vi "Configure Scale Band IO.vi"(0 "VISA resource name":refnum<visa-resource-name>, 1 "Lower Position (In Log Calc) (1.00E+0)":dbl=1.0 format="%.2e", 2 "Upper Position (In Log Calc) (1.00E+2)":dbl=100.0 format="%.2e", 5 "Channel (0001)":string="0001", 7 "Area (0 : Off)":i32(ring) items=["Off", "In", "Out"], 9 "Color":cluster{"R":i32, "G":i32, "B":i32} {"B" min=0 max=255 step=1; "G" min=0 max=255 step=1; "R" min=0 max=255 step=1}, 11 "error in (no error)":errorcluster, 12 "Lower Position (0)":i32, 13 "Upper Position (1)":i32=1) -> (4 "VISA resource name out":refnum<visa-resource-name>, 6 "Channel":string, 15 "error out":errorcluster)   [LabVIEW 2020, in "Yokogawa GX Series.lvlib"]
doc: "Sets the green band of IO channel.\n\nCommand: SBandIO"
uses:
  <instrlib>/Yokogawa GX Series/Yokogawa GX Series.lvlib
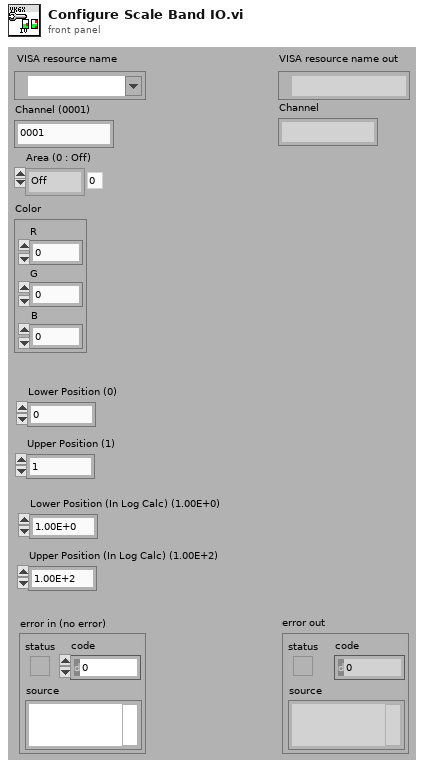
[diagram p1: front panel]
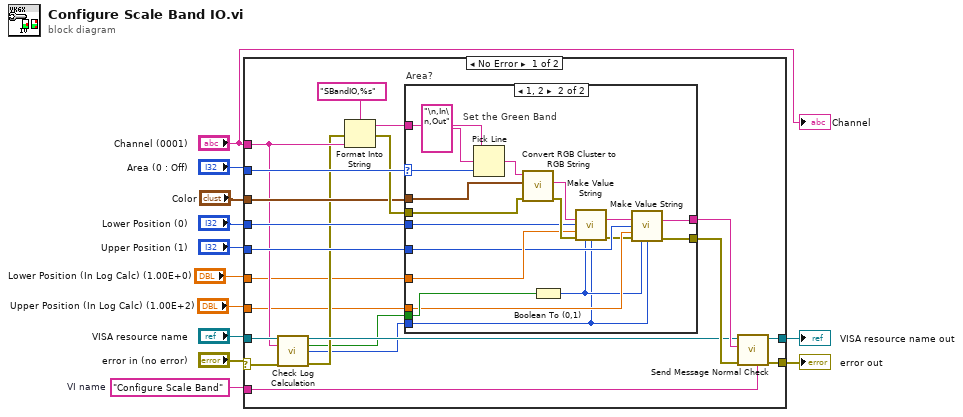
[diagram p0: block diagram]
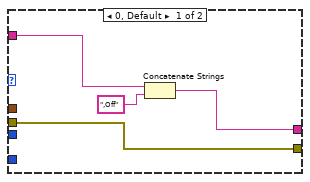
[diagram p2: hidden frame]
diagram:
  w12 = "Configure Scale Band"  # VI name
  n1 = case shown="No Error" "error in (no error)" {
    selector: "error in (no error)" -> [w21 w57]
    tunnel: w12 -> [w32 _]
    tunnel: "Area (0 : Off)" -> [w31 _]
    tunnel: "Lower Position (0)" -> [w28 _]
    tunnel: "Upper Position (1)" -> [w27 _]
    tunnel: "VISA resource name" -> [w20 w58]
    tunnel: [w24 w58] -> w7
    tunnel: [w23 w57] -> w6
    tunnel: "Color" -> [w22 _]
    tunnel: "Channel (0001)" -> [w19 _]
    tunnel: "Lower Position (In Log Calc) (1.00E+0)" -> [w16 _]
    tunnel: "Upper Position (In Log Calc) (1.00E+2)" -> [w15 _]
    frame No Error {
      n2 = call <instrlib>:"Check Log Calculation.vi"("VISA resource name"=w20, "Channel (0001)"=w19, "error in (no error)"=w21) -> ("VISA resource name out"=w18:refnum<visa-resource-name>, "Result"=w14:bool, "Float Position"=w13:i32, "error out"=w17:errorcluster)  [unwired: 9 in]
      n3 = Format Into String(format string="SBandIO,%s", error in=w17, w19) -> (resulting string=w26:string, error out=w30:errorcluster)  [unwired: 1 in]
      n4 = case "Area?" shown="1, 2" w31 {
        selector: w31 -> [_ w55]
        tunnel: w30 -> [w37 w52]
        tunnel: [w37 w41] -> w29
        tunnel: w28 -> [_ w48]
        tunnel: w27 -> [_ w44]
        tunnel: [w34 w40] -> w25
        tunnel: w26 -> [w35 w54]
        tunnel: w22 -> [_ w53]
        tunnel: w16 -> [_ w47]
        tunnel: w15 -> [_ w43]
        tunnel: w14 -> [_ w46]
        tunnel: w13 -> [_ w38]
        frame 0, Default {
          n5 = Concatenate Strings(w35, ",Off") -> (w34:string)
        }
        frame 1, 2 {
          # "Set the Green Band"
          n6 = Pick Line(string ("")=w54, multi-line string="\n,In\n,Out" ("形式文字列"), line index=w55) -> (output string=w51:string)
          n7 = call <instrlib>:"Convert RGB Cluster to RGB String.vi"("error in (no error)"=w52, "RGB"=w53, "Initial String"=w51) -> ("error out"=w50:errorcluster, "RGB String"=w49:string)  [unwired: 7 in]
          n8 = Boolean To (0,1)(Boolean=w46) -> (0, 1=w39:i16)
          n9 = call <instrlib>:"Make Value String.vi"("Initial String (\"\")"=w49, "Int Value (0)"=w48, "Float Value (0)"=w47, "Error In"=w50, "Kind Of Value (0: Int)"=w39, "Float Decimal Position (1)"=w38) -> ("Resulting String"=w45:string, "Error Out"=w42:errorcluster)  [unwired: 8 in]
          n10 = call <instrlib>:"Make Value String.vi"("Initial String (\"\")"=w45, "Int Value (0)"=w44, "Float Value (0)"=w43, "Error In"=w42, "Kind Of Value (0: Int)"=w39, "Float Decimal Position (1)"=w38) -> ("Resulting String"=w40:string, "Error Out"=w41:errorcluster)  [unwired: 8 in]
        }
      }
      n11 = call <instrlib>:"Send Message Normal Check.vi"("Source (\"\")"=w32, "error in (no error)"=w29, "Send Message (\"\")"=w25, "VISA resource name"=w18) -> ("error out"=w23:errorcluster, "VISA resource name out"=w24:refnum<visa-resource-name>)  [unwired: 2 in, 4 out]
    }
    frame Error {
    }
  }
  "error out" <- w6
  "VISA resource name out" <- w7
  "Channel" <- "Channel (0001)"
